vi "camera_multiple_image_test.vi"() -> ()   [LabVIEW 2019]
panel:
  out "Error Out":errorcluster
  in  "ExposureTime_us":u32
  in  "stop":bool
  in  "Retake":bool
  out "Image":T1(plugin-control)
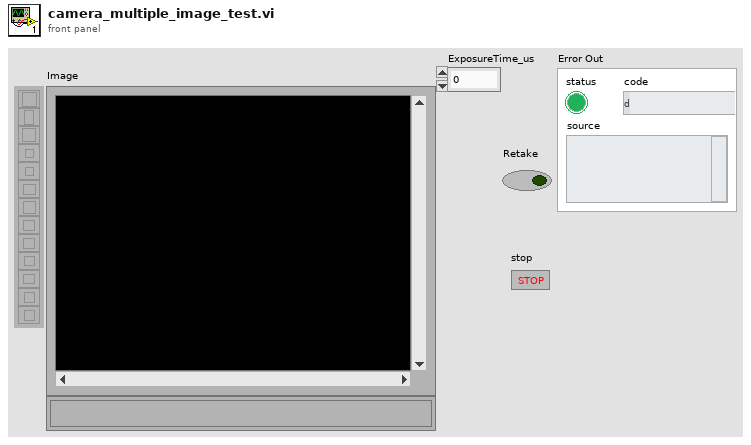
[diagram p1: front panel]
types:
  T1 = typedef "IMAQ Image.ctl" = refnum<image>
  T2 = typedef "Image Type" = u32
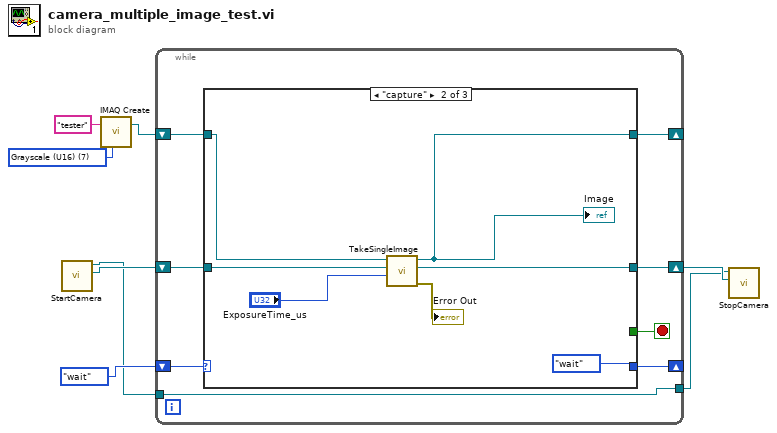
[diagram p0: block diagram]
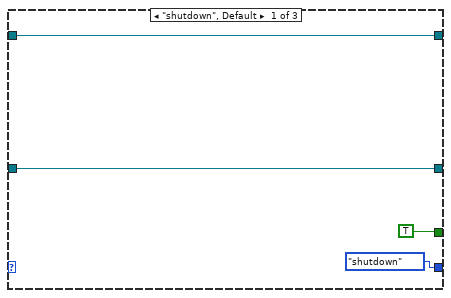
[diagram p2: hidden frame]
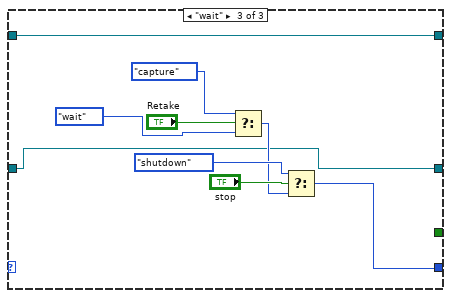
[diagram p3: hidden frame]
diagram:
  w1 = T2 7 items=["Grayscale (U8)", "Grayscale (I16)", "Grayscale (SGL)", "Complex (CSG)", "RGB (U32)", "HSL (U32)", "RGB (U64)", "Grayscale (U16)"] ("Image Type")
  n1 = call "StartCamera.vi"() -> ("TLCamera reference out"=w7:refnum<k24>, "TLCameraSDK reference out"=w4:refnum<k24>)  [unwired: 9 in, 1 out]
  n2 = call "IMAQ Create"("Image Name"="tester", "Image Type"=w1) -> ("New Image"=w3:T1)  [unwired: 3 in, 1 out]
  n3 = while {
    shift-right: [w15] -> _
    shift-left: enum16{"shutdown", "capture", "wait"}."wait" -> [w16]
    shift-right: [w14] -> _
    shift-left: w3 -> [w10]
    shift-right: [w12] -> w6
    shift-left: w7 -> [w13]
    tunnel: [w11] -> w5
    tunnel: w4 -> [w11]
    stop <- w9 stop-if-true
    n4 = case shown="\"capture\"" w16 {
      tunnel: [enum16{"shutdown", "capture", "wait"}."shutdown" enum16{"shutdown", "capture", "wait"}."wait" w30] -> w15
      tunnel: [w20 w27 w29] -> w14
      tunnel: w13 -> [w19 w26 w28]
      tunnel: [w19 w24 w28] -> w12
      tunnel: w10 -> [w20 w23 w29]
      tunnel: [TRUE _ _] -> w9
      frame "shutdown", Default {
      }
      frame "capture" {
        n5 = call "TakeSingleImage.vi"("Image"=w23, "TLCamera reference in"=w26, "ExposureTime_us"="ExposureTime_us") -> ("Image Out"=w27:T1, "TLCamera reference out"=w24:refnum<k24>, "Error Out"=→"Error Out":errorcluster)  [unwired: 5 in]
        "Image" <- w27
      }
      frame "wait" {
        n6 = Select(t=enum16{"shutdown", "capture", "wait"}."capture", s="Retake", f=enum16{"shutdown", "capture", "wait"}."wait") -> (s? t:f=w34:enum16{"shutdown", "capture", "wait"})
        n7 = Select(t=enum16{"shutdown", "capture", "wait"}."shutdown", s="stop", f=w34) -> (s? t:f=w30:enum16{"shutdown", "capture", "wait"})
      }
    }
  }
  n8 = call "StopCamera.vi"("TLCamera reference"=w6, "TLCameraSDK reference"=w5) -> ()  [unwired: 9 in, 1 out]
